vi "Test 1.vi"() -> ()   [LabVIEW 2012]
uses:
  WT1600/WT1600/WT1600.lvclass
  <vilib>/ActorFramework/Message Queue/Message Queue.lvclass/Message Queue.ctl
  <vilib>/ActorFramework/Message Enqueuer/Message Enqueuer.lvclass/Message Enqueuer.ctl
  <vilib>/ActorFramework/Message Enqueuer/Enqueue.vi
  Global VI.vi
  <vilib>/ActorFramework/Message Priority Queue/Priority Enqueue.vi
  <vilib>/ActorFramework/Stop Msg/Stop Msg.lvclass
  <vilib>/ActorFramework/Actor/Actor.lvclass
  <vilib>/ActorFramework/Message Queue/Message Queue.lvclass
panel:
  out "error out 2":errorcluster
  out "error out":errorcluster
  in  "VISA WT1600":refnum<visa-resource-name>="GPIB0::1::INSTR"
  in  "stop":bool
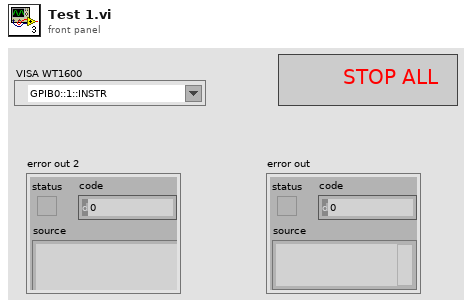
[diagram p1: front panel]
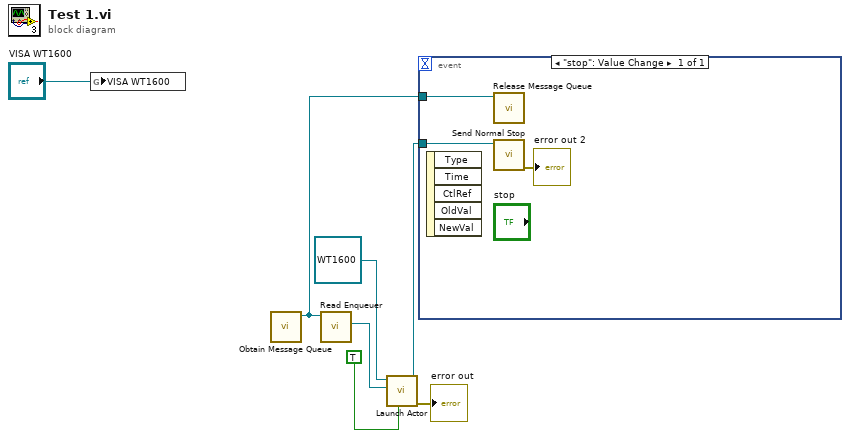
[diagram p0: block diagram]
diagram:
  n1 = global write "Global VI.vi" "VISA WT1600"("VISA WT1600") -> ()
  n2 = call <vilib>:"Obtain Message Queue.vi"() -> ("Message Queue"=w6:refnum<class "Message Queue.lvclass">)  [unwired: 10 in, 1 out]
  n3 = call <vilib>:"Read Enqueuer.vi"("Message Queue"=w6) -> ("Message Enqueuer"=w7:refnum<class "Message Enqueuer.lvclass">)  [unwired: 10 in]
  n4 = call <vilib>:"Launch Actor.vi"("Open Actor Core front panel? (F)"=TRUE, "Actor-to-Caller Enqueuer"=w7, "Actor"=refnum<class "WT1600.lvclass"> refnum ("WT1600.lvlib:WT1600.lvclass")) -> ("error out"=→"error out":errorcluster, "Caller-To-Actor Enqueuer"=w1:refnum<class "Message Enqueuer.lvclass">)  [unwired: 7 in]
  n5 = event shown="[0] \"stop\": Value Change" {
    selector: _ -> [_]
    dyn-events: _ -> [_]
    timeout: _ -> [_]
    tunnel: w1 -> [w10]
    tunnel: w6 -> [w9]
    event "stop": Value Change {
      n6 = event-data() -> ()  [unwired: 1 in, 5 out]
      n7 = call <vilib>:"Release Message Queue.vi"("Message Queue"=w9) -> ()  [unwired: 9 in, 2 out]
      n8 = call <vilib>:"Send Normal Stop.vi"("Message Enqueuer"=w10) -> ("error out"=→"error out 2":errorcluster)  [unwired: 10 in]
    }
  }
